vi "CRON_Example.vi"() -> ()   [LabVIEW 2024]
uses:
  CRON.lvclass
  C:/Git/JA/JQMH/RQMHCore/ModuleCore/Module.lvclass
  C:/Git/JA/JQMH/ModuleTemplates/CRON/CRON.lvclass
  RQMHCore/ModuleCore/Module.lvclass
  <vilib>/LabVIEW Open Source Project/Cron Scheduler/Cron.Unix/Cron.Unix.lvclass
  <vilib>/LabVIEW Open Source Project/Cron Scheduler/Cron.Quartz/Cron.Quartz.lvclass
panel:
  in  "Schedule 3":string="* * * * *"
  out "Time 3":u32
  out "Time 2":u32
  in  "Schedule 2":string="* * * * *"
  in  "Schedule":string="* * * * *"
  out "Time":u32
  # "https://crontab.cronhub.io/"
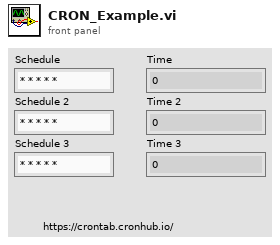
[diagram p1: front panel]
types:
  T1 = typedef "Module.lvclass/StandardBroadcasts.ctl" = cluster{"Died":refnum<user-event>, "Started":refnum<user-event>}
  T2 = typedef "CRON.lvclass/Broadcast Events--cluster.ctl" = cluster{"Stopped":refnum<user-event>, "Fired":refnum<user-event>}
  T3 = typedef "CRON.lvclass/Stopped.ctl" = bool
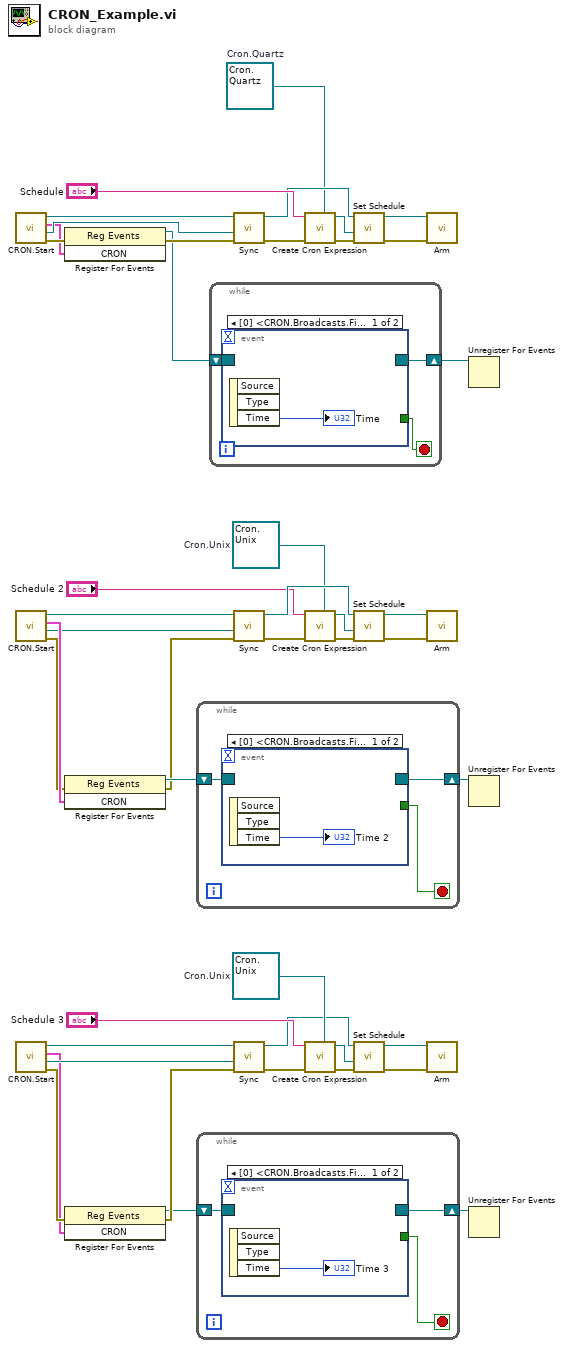
[diagram p0: block diagram]
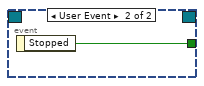
[diagram p2: hidden frame]
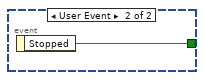
[diagram p3: hidden frame]
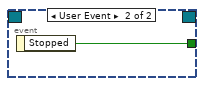
[diagram p4: hidden frame]
diagram:
  w1 = refnum<class "Cron.Quartz.lvclass"> refnum  # Cron.Quartz
  w6 = refnum<class "Cron.Unix.lvclass"> refnum  # Cron.Unix
  w27 = refnum<class "Cron.Unix.lvclass"> refnum  # Cron.Unix
  n1 = call "CRON.Start.vi"() -> ("error out"=w43:errorcluster, "StartupHandshake out"=w44:refnum<class "ModuleStartup.lvclass">, "CRON"=w39:cluster{"Broadcasts":T1, "Broadcasts":T2}, "NewTemplate out"=w45:refnum<class "CRON.lvclass">)  [unwired: 8 in]
  n2 = call "CRON.Start.vi"() -> ("error out"=w19:errorcluster, "StartupHandshake out"=w18:refnum<class "ModuleStartup.lvclass">, "CRON"=w23:cluster{"Broadcasts":T1, "Broadcasts":T2}, "NewTemplate out"=w17:refnum<class "CRON.lvclass">)  [unwired: 8 in]
  n3 = call "CRON.Start.vi"() -> ("error out"=w14:errorcluster, "StartupHandshake out"=w15:refnum<class "ModuleStartup.lvclass">, "CRON"=w10:cluster{"Broadcasts":T1, "Broadcasts":T2}, "NewTemplate out"=w16:refnum<class "CRON.lvclass">)  [unwired: 8 in]
  n4 = register-events(error in=w43, w39) -> (reference out=w41:refnum<event-registration>, error out=w42:errorcluster)  [unwired: 1 in]
  n5 = register-events(error in=w19, w23) -> (reference out=w21:refnum<event-registration>, error out=w20:errorcluster)  [unwired: 1 in]
  n6 = register-events(error in=w14, w10) -> (reference out=w12:refnum<event-registration>, error out=w13:errorcluster)  [unwired: 1 in]
  n7 = while {
    shift-right: [w48] -> w22
    shift-left: w21 -> [w47]
    stop <- w46 stop-if-true
    n8 = event shown="[0] <CRON.Broadcasts.Fired>: User Event" {
      selector: w47 -> [_ _]
      dyn-events: [_ _] -> w48
      timeout: _ -> [_ _]
      tunnel: [_ w50] -> w46
      event User Event {
        n9 = event-data() -> ("Time"=→"Time 2":u32)  [unwired: 1 in, 2 out]
      }
      event User Event {
        n10 = event-data() -> ("Stopped"=w50:T3)  [unwired: 1 in]
      }
    }
  }
  n11 = while {
    shift-right: [w53] -> w11
    shift-left: w12 -> [w52]
    stop <- w51 stop-if-true
    n12 = event shown="[0] <CRON.Broadcasts.Fired>: User Event" {
      selector: w52 -> [_ _]
      dyn-events: [_ _] -> w53
      timeout: _ -> [_ _]
      tunnel: [_ w55] -> w51
      event User Event {
        n13 = event-data() -> ("Time"=→"Time 3":u32)  [unwired: 1 in, 2 out]
      }
      event User Event {
        n14 = event-data() -> ("Stopped"=w55:T3)  [unwired: 1 in]
      }
    }
  }
  n15 = while {
    shift-right: [w57] -> w40
    shift-left: w41 -> [w58]
    stop <- w56 stop-if-true
    n16 = event shown="[0] <CRON.Broadcasts.Fired>: User Event" {
      selector: w58 -> [_ _]
      dyn-events: [_ _] -> w57
      timeout: _ -> [_ _]
      tunnel: [_ w60] -> w56
      event User Event {
        n17 = event-data() -> ("Time"=→"Time":u32)  [unwired: 1 in, 2 out]
      }
      event User Event {
        n18 = event-data() -> ("Stopped"=w60:T3)  [unwired: 1 in]
      }
    }
  }
  n19 = call "Sync.vi"("error in (no error)"=w42, "StartupHandshake out"=w44, "JQMHCore in"=w45) -> ("error out"=w32:errorcluster, "JQMHCore out"=w35:refnum<class "CRON.lvclass">)  [unwired: 7 in]
  n20 = call "Sync.vi"("error in (no error)"=w20, "StartupHandshake out"=w18, "JQMHCore in"=w17) -> ("error out"=w31:errorcluster, "JQMHCore out"=w28:refnum<class "CRON.lvclass">)  [unwired: 7 in]
  n21 = call "Sync.vi"("error in (no error)"=w13, "StartupHandshake out"=w15, "JQMHCore in"=w16) -> ("error out"=w2:errorcluster, "JQMHCore out"=w5:refnum<class "CRON.lvclass">)  [unwired: 7 in]
  n22 = call <vilib>:"Create Cron Expression.vi"("Cron in"=w1, "error in (no error)"=w32, "Cron Expression"="Schedule") -> ("error out"=w37:errorcluster, "Cron out"=w38:refnum<class "Cron.Quartz.lvclass">)  [unwired: 6 in, 1 out]
  n23 = call <vilib>:"Create Cron Expression.vi"("Cron in"=w27, "error in (no error)"=w31, "Cron Expression"="Schedule 2") -> ("error out"=w25:errorcluster, "Cron out"=w24:refnum<class "Cron.Unix.lvclass">)  [unwired: 6 in, 1 out]
  n24 = call <vilib>:"Create Cron Expression.vi"("Cron in"=w6, "error in (no error)"=w2, "Cron Expression"="Schedule 3") -> ("error out"=w8:errorcluster, "Cron out"=w9:refnum<class "Cron.Unix.lvclass">)  [unwired: 6 in, 1 out]
  n25 = call "Set Schedule.vi"("error in (no error)"=w37, "Cron"=w38, "module in"=w35) -> ("error out"=w33:errorcluster, "module out"=w34:refnum<class "CRON.lvclass">)  [unwired: 6 in, 1 out]
  n26 = call "Set Schedule.vi"("error in (no error)"=w25, "Cron"=w24, "module in"=w28) -> ("error out"=w30:errorcluster, "module out"=w29:refnum<class "CRON.lvclass">)  [unwired: 6 in, 1 out]
  n27 = call "Set Schedule.vi"("error in (no error)"=w8, "Cron"=w9, "module in"=w5) -> ("error out"=w3:errorcluster, "module out"=w4:refnum<class "CRON.lvclass">)  [unwired: 6 in, 1 out]
  n28 = call "Arm.vi"("error in (no error)"=w33, "module in"=w34) -> ()  [unwired: 7 in, 3 out]
  n29 = call "Arm.vi"("error in (no error)"=w30, "module in"=w29) -> ()  [unwired: 7 in, 3 out]
  n30 = call "Arm.vi"("error in (no error)"=w3, "module in"=w4) -> ()  [unwired: 7 in, 3 out]
  n31 = Unregister For Events(event registration refnum=w40) -> ()  [unwired: 1 in, 1 out]
  n32 = Unregister For Events(event registration refnum=w22) -> ()  [unwired: 1 in, 1 out]
  n33 = Unregister For Events(event registration refnum=w11) -> ()  [unwired: 1 in, 1 out]
